vi "SECoP-updateParameter.vi"(6 "Timestamp":dbl=nan, 7 "sigma (SECoP_data)":T1 {"ptr64" format="%.0x"; "ptr32" format="%.0x"}, 8 "error in (no error)":errorcluster, 9 "value (SECoP_data)":T1 {"ptr64" format="%.0x"; "ptr32" format="%.0x"}, 10 "parameter name":string, 11 "DLL path (in)":T2) -> (0 "error out":errorcluster, 3 "DLL path (out)":T2)   [LabVIEW 2023, in "SECoP.lvlib"]
doc: "Call <b>\"SECoP-updateParameter.vi\"</b>, if you have a new value for an existing parameter (read- or writable). All clients which subscribed to this module should be informed about the new value..\n\n<b>DLL path</b> input and output of cluster from \"SECoP-Initialize.vi\"\n<b>parameter name</b> full name of parameter including node id and module name (format <b>node-id:module:parameter</b>)\n<b>value (SECoP_data)</b> new value of parameter\n<b>sigma (SECoP_data)</b> if applicable, the error bar of the new value of parameter\n<b>timestamp</b> time in seconds (with fraction) from 1970/1/1 0:0am of data (or NaN for actual time)"
uses:
  SECoP.lvlib
  SECoP-libraries.ctl
  SECoP-data/SECoP-data.ctl
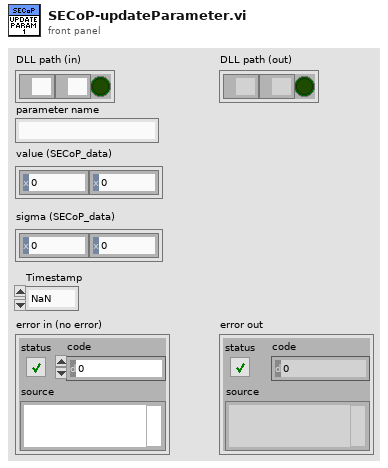
[diagram p1: front panel]
types:
  T1 = typedef "SECoP.lvlib/SECoP-data.ctl" = cluster{"ptr32":u32, "ptr64":u64}
  T2 = typedef "SECoP.lvlib/SECoP-libraries.ctl" = cluster{"serverDLL":path, "variantDLL":path, "cleanup_mode":bool}
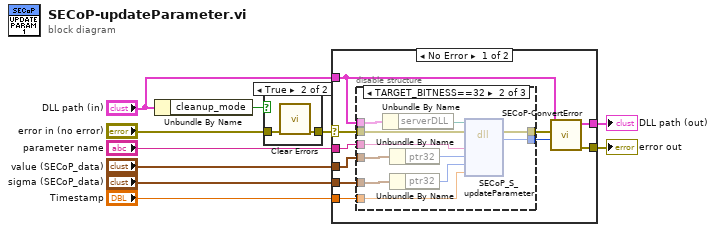
[diagram p0: block diagram]
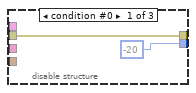
[diagram p3: hidden frame]
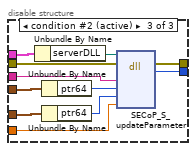
[diagram p4: hidden frame]
diagram:
  n1 = Unbundle By Name("DLL path (in)") -> ("cleanup_mode"=w7:bool)
  n2 = case shown="True" w7 {
    tunnel: "error in (no error)" -> [w11 w13]
    tunnel: [w11 w12] -> w5
    frame False {
    }
    frame True {
      n3 = call <vilib>:"Clear Errors.vi"("error in (no error)"=w13) -> ("error out"=w12:errorcluster)  [unwired: 5 in, 1 out]
    }
  }
  n4 = case shown="No Error" w5 {
    selector: w5 -> [w19 w48]
    tunnel: "DLL path (in)" -> [w14 w49]
    tunnel: [w22 w49] -> w10
    tunnel: [w23 w48] -> w9
    tunnel: "parameter name" -> [w18 _]
    tunnel: "Timestamp" -> [w17 _]
    tunnel: "value (SECoP_data)" -> [w16 _]
    tunnel: "sigma (SECoP_data)" -> [w15 _]
    frame No Error {
      n5 = disable-structure shown="TARGET_BITNESS==32" {
        disable-tunnel: [w25 w36 w47] -> w21
        disable-tunnel: [-20 w35 w46] -> w20
        disable-tunnel: w14 -> [_ w34 w45]
        disable-tunnel: w19 -> [w25 w33 w44]
        disable-tunnel: w18 -> [_ w32 w43]
        disable-tunnel: w17 -> [_ w31 w42]
        disable-tunnel: w16 -> [_ w30 w41]
        disable-tunnel: w15 -> [_ w28 w39]
        frame condition #0 {
        }
        frame condition #1 {
          n6 = Unbundle By Name(w34) -> ("serverDLL"=w26:path)
          n7 = Unbundle By Name(w30) -> ("ptr32"=w29:u32)
          n8 = Unbundle By Name(w28) -> ("ptr32"=w27:u32)
          n9 = dll-call lib="Z:/Praktische Aufgaben/SECoP-LabVIEW2015/32bit/SECoP32.dll" fn="SECoP_S_updateParameter"(path in=w26, error in=w33, "ParameterName"=w32, "value"=w29, "sigma"=w27, "Timestamp"=w31) -> (error out=w36:errorcluster, "return type"=w35:i32)  [unwired: 5 in, 1 out]
        }
        frame condition #2 (active) {
          n10 = Unbundle By Name(w45) -> ("serverDLL"=w37:path)
          n11 = Unbundle By Name(w41) -> ("ptr64"=w40:u64)
          n12 = Unbundle By Name(w39) -> ("ptr64"=w38:u64)
          n13 = dll-call lib="Z:/Praktische Aufgaben/SECoP-LabVIEW2015/32bit/SECoP32.dll" fn="SECoP_S_updateParameter"(path in=w37, error in=w44, "ParameterName"=w43, "value"=w40, "sigma"=w38, "Timestamp"=w42) -> (error out=w47:errorcluster, "return type"=w46:i32)  [unwired: 5 in, 1 out]
        }
      }
      n14 = call "SECoP-ConvertError.vi"("return code"=w20, "error in (no error)"=w21, "DLL path (in)"=w14) -> ("error out"=w23:errorcluster, "DLL path (out)"=w22:T2)  [unwired: 7 in]
    }
    frame Error {
    }
  }
  "DLL path (out)" <- w10
  "error out" <- w9
